vi "MultiChannelfFeedbackCooling (FPGA)_PIDXYZ.vi"() -> ()   [LabVIEW 2016]
doc: "This VI will read single point values from 4 channels of a R Series board at a specified rate."
uses:
  <vilib>/rvi/Emulation/niFpgaGetClockAttributes.vi
  <vilib>/rvi/Emulation/niFpgaSctlEmulationGetInTimedLoop.vi
  <vilib>/rvi/Emulation/niFpgaEmulationReportErrorSimple.vi
  <vilib>/rvi/eio/common/nirviEmuTemplateMethod_errors.vi
  <vilib>/rvi/Memory/Memory_Emulation/nirvimemoryFastEmulation.vi
  <vilib>/rvi/Memory/Memory_Emulation/nirvimemoryEmulation.vi
  <vilib>/rvi/Emulation/niFpgaEmulationIsFPGAContextNoSignature.vi
  <vilib>/rvi/DataTransferAndStorage/Container/Common/niFpgaContainerGetUniqueNameForEmu.vi
  <vilib>/rvi/Emulation/niFpgaProcessEmulError.vi
  <vilib>/rvi/errors/nirviReportUnexpectedCaseInternalError (U32).vi
  <vilib>/rvi/Memory/Memory_Emulation/niFpgaMemoryEmulationCacheClearOnFirstRun.vi
  <vilib>/rvi/Memory/Memory_Emulation/nirvimemoryEmulationManagerCache_MakeExclusive.vi
  <vilib>/rvi/Memory/Memory_Emulation/niFpgaMemoryEmulationValidateCache.vi
  <vilib>/rvi/Memory/Memory_Emulation/nirvimemoryEmulationManagerCache_InsertValue.vi
  <vilib>/Utility/error.llb/Clear Errors.vi
  <vilib>/rvi/Memory/Memory_Emulation/nirvimemoryEmulationManagerCache_ReleaseExclusive.vi
  <vilib>/rvi/Memory/Memory_Emulation/nirvimemoryEmulationManagerCache_GetValue.vi
  <vilib>/rvi/Memory/Memory_Emulation/nirvimemoryEmulationManagerCache_SetValue.vi
  <vilib>/rvi/Emulation/niFpgaSctlEmulationResourceMgr.vi
  <vilib>/rvi/Emulation/niFpgaCriticalErrorInLSC.vi
  <vilib>/eio/EIONode/EIONode.xnode
  <vilib>/rvi/DataTransferAndStorage/Container/XNode/niFpgaContainer.xnode
  <vilib>/rvi/FXPMathLib/FxpInterpret/XNode/nifxpmath_Interpret.xnode
panel:
  in  "EOM_offset":i16
  in  "EOM_seed":u32=4294967295 caption="seed"
  in  "EOM reset":bool caption="reset"
  in  "EOM_threshold":i16
  in  "EOM_amplitude":i16
  in  "hp coeff band imgZ":i32[](array[numeric])=[-850883994, 1909449570, 958518847, -975456236, 2033039520, 1020559395]
  in  "lp coeff band imgZ":i32[](array[numeric])=[-955995012, 2025731616, 1001305, -1023351008, 2092954700, 1034533]
  in  "hp coeff band dZ":i32[](array[numeric])=[-850883994, 1909449570, 958518847, -975456236, 2033039520, 1020559395]
  in  "lp coeff band dZ":i32[](array[numeric])=[-955995012, 2025731616, 1001305, -1023351008, 2092954700, 1034533]
  in  "lp coeff band Z":i32[](array[numeric])=[-955995012, 2025731616, 1001305, -1023351008, 2092954700, 1034533]
  in  "hp coeff band Z":i32[](array[numeric])=[-850883994, 1909449570, 958518847, -975456236, 2033039520, 1020559395]
  in  "lp coeff band Y":i32[](array[numeric])=[-955995012, 2025731616, 1001305, -1023351008, 2092954700, 1034533]
  in  "hp coeff band Y":i32[](array[numeric])=[-850883994, 1909449570, 958518847, -975456236, 2033039520, 1020559395]
  in  "lp coeff band X":i32[](array[numeric])=[-955995012, 2025731616, 1001305, -1023351008, 2092954700, 1034533]
  in  "hp coeff band X":i32[](array[numeric])=[-850883994, 1909449570, 958518847, -975456236, 2033039520, 1020559395]
  in  "dg band dZ":fxp<+/-,24,12>
  in  "dg band imgZ":fxp<+/-,24,12>
  in  "dg band Z":fxp<+/-,24,12>
  in  "dg band Y":fxp<+/-,24,12>
  in  "dg band X":fxp<+/-,24,12>
  in  "lp coeff band X":i32[](array[numeric])=[1008310688, 32715568]
  in  "pg 1":fxp<+/-,24,12>
  in  "ig 1":fxp<+/-,24,6>
  in  "pg 0":fxp<+/-,24,12>
  in  "ig 0":fxp<+/-,24,6>
  in  "pg_img":fxp<+/-,24,12>
  in  "dg_img":fxp<+/-,24,12>
  in  "ig_img":fxp<+/-,24,6>
  in  "setpt_img":i16
  out "AI_img":i16
  in  "lp coeff_img":i32[](array[numeric])=[1008310688, 32715568]
  in  "Upper lim_img":fxp<+/-,16,16>
  in  "Lower lim_img":fxp<+/-,16,16>
  in  "lp coeff d2":i32[](array[numeric])=[1008310688, 32715568]
  in  "hp coeff_img":i32[](array[numeric])=[946630756, 1010186290]
  out "tot_fb_img":i16
  out "fb_img":i16
  in  "output offset_img":i16
  in  "lp coeff 2":i32[](array[numeric])=[1008310688, 32715568]
  in  "data_buffer3":i16
  in  "Arb gain (ch2)":fxp<+/-,24,12>=0.5 caption="RMS"
  in  "lp coeff 0":i32[](array[numeric])=[1008310688, 32715568]
  in  "lp coeff 1":i32[](array[numeric])=[1008310688, 32715568]
  in  "hp coeff d2":i32[](array[numeric])=[946630756, 1010186290]
  in  "hp coeff 2":i32[](array[numeric])=[946630756, 1010186290]
  in  "hp coeff 1":i32[](array[numeric])=[946630756, 1010186290]
  in  "hp coeff 0":i32[](array[numeric])=[946630756, 1010186290]
  in  "Use_PID2_X 2":bool
  out "AI5":i16
  in  "Dc Pos d2":i16
  out "tot_fb_2":i16
  out "tot_fb_1":i16
  out "tot_fb_0":i16
  out "fb_d2":i16
  in  "output offset 2":i16
  in  "output offset 1":i16
  in  "output offset 0":i16
  in  "Lower lim 4":fxp<+/-,16,16>
  in  "Upper lim d0 3":fxp<+/-,16,16>
  in  "pg d0 3":fxp<+/-,24,12>
  in  "ig d03":fxp<+/-,24,6>
  in  "dg d0 3":fxp<+/-,24,12>
  out "fb_2":i16
  in  "ig 3":fxp<+/-,24,6>
  out "written_address":u32
  in  "ready_to_write":bool
  in  "Arb steps per cycle":u16
  in  "data_buffer2":i16
  in  "data_buffer_1":i16
  in  "write_address":u16
  in  "Arb gain (ch1)":fxp<+/-,24,12>=0.5 caption="RMS"
  in  "Arb gain (ch0)":fxp<+/-,24,12>=0.5 caption="RMS"
  out "fb_1":i16
  out "fb_0":i16
  in  "Dc Pos 1":i16
  in  "Dc Pos 0":i16
  in  "Lower lim 2":fxp<+/-,16,16>
  in  "Upper lim 2":fxp<+/-,16,16>
  in  "dg 2":fxp<+/-,24,12>
  in  "pg 2":fxp<+/-,24,12>
  out "AI2":i16
  in  "Dc Pos 2":i16
  out "AI1":i16
  in  "dg 1":fxp<+/-,24,12>
  in  "Upper lim 1":fxp<+/-,16,16>
  in  "Lower lim 1":fxp<+/-,16,16>
  out "AI0":i16
  in  "dg 0":fxp<+/-,24,12>
  in  "Upper lim 0":fxp<+/-,16,16>
  in  "Lower lim 0":fxp<+/-,16,16>
  in  "Count(uSec)":u32
  out "FPGA Error Out":errorcluster
  in  "Stop":bool
  # "test"
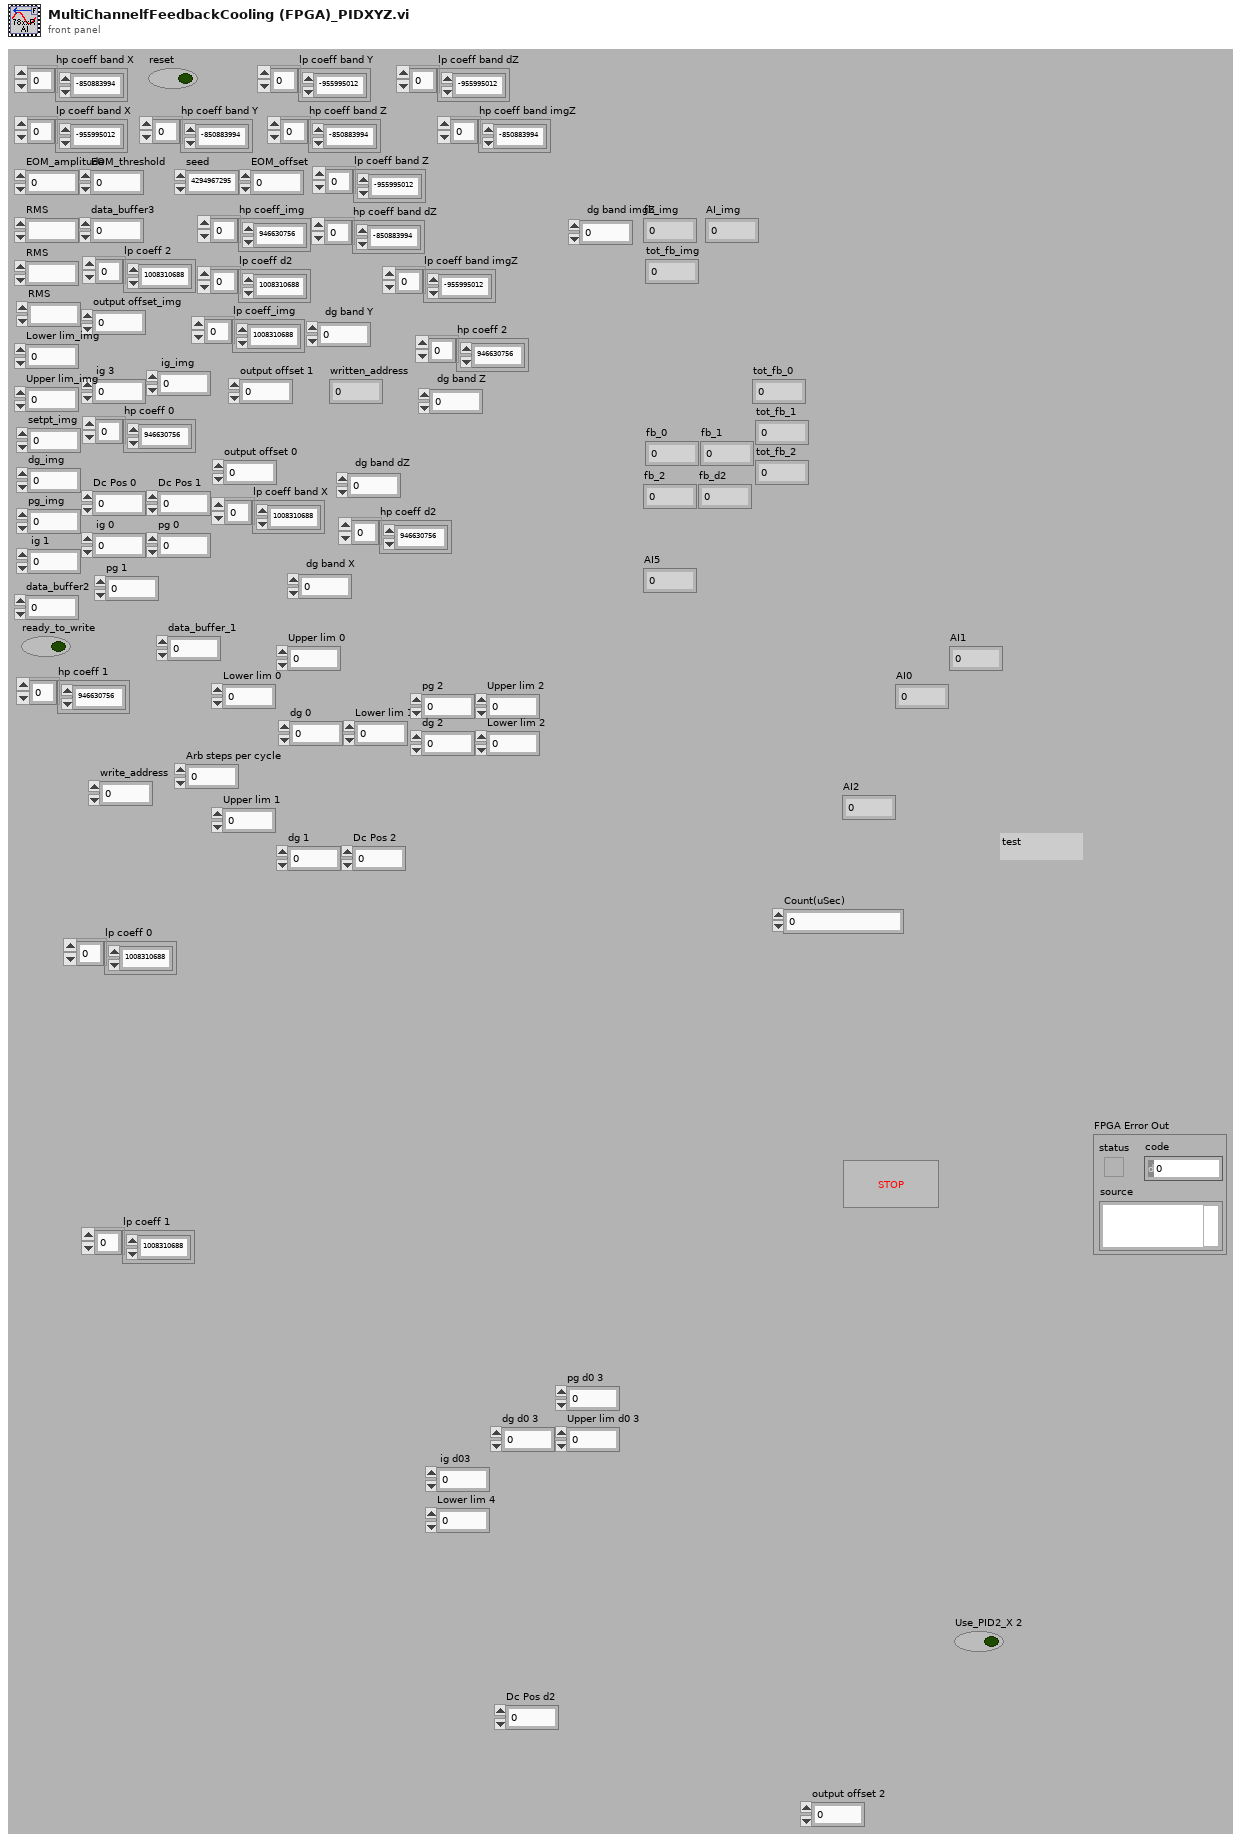
[diagram p1: front panel]
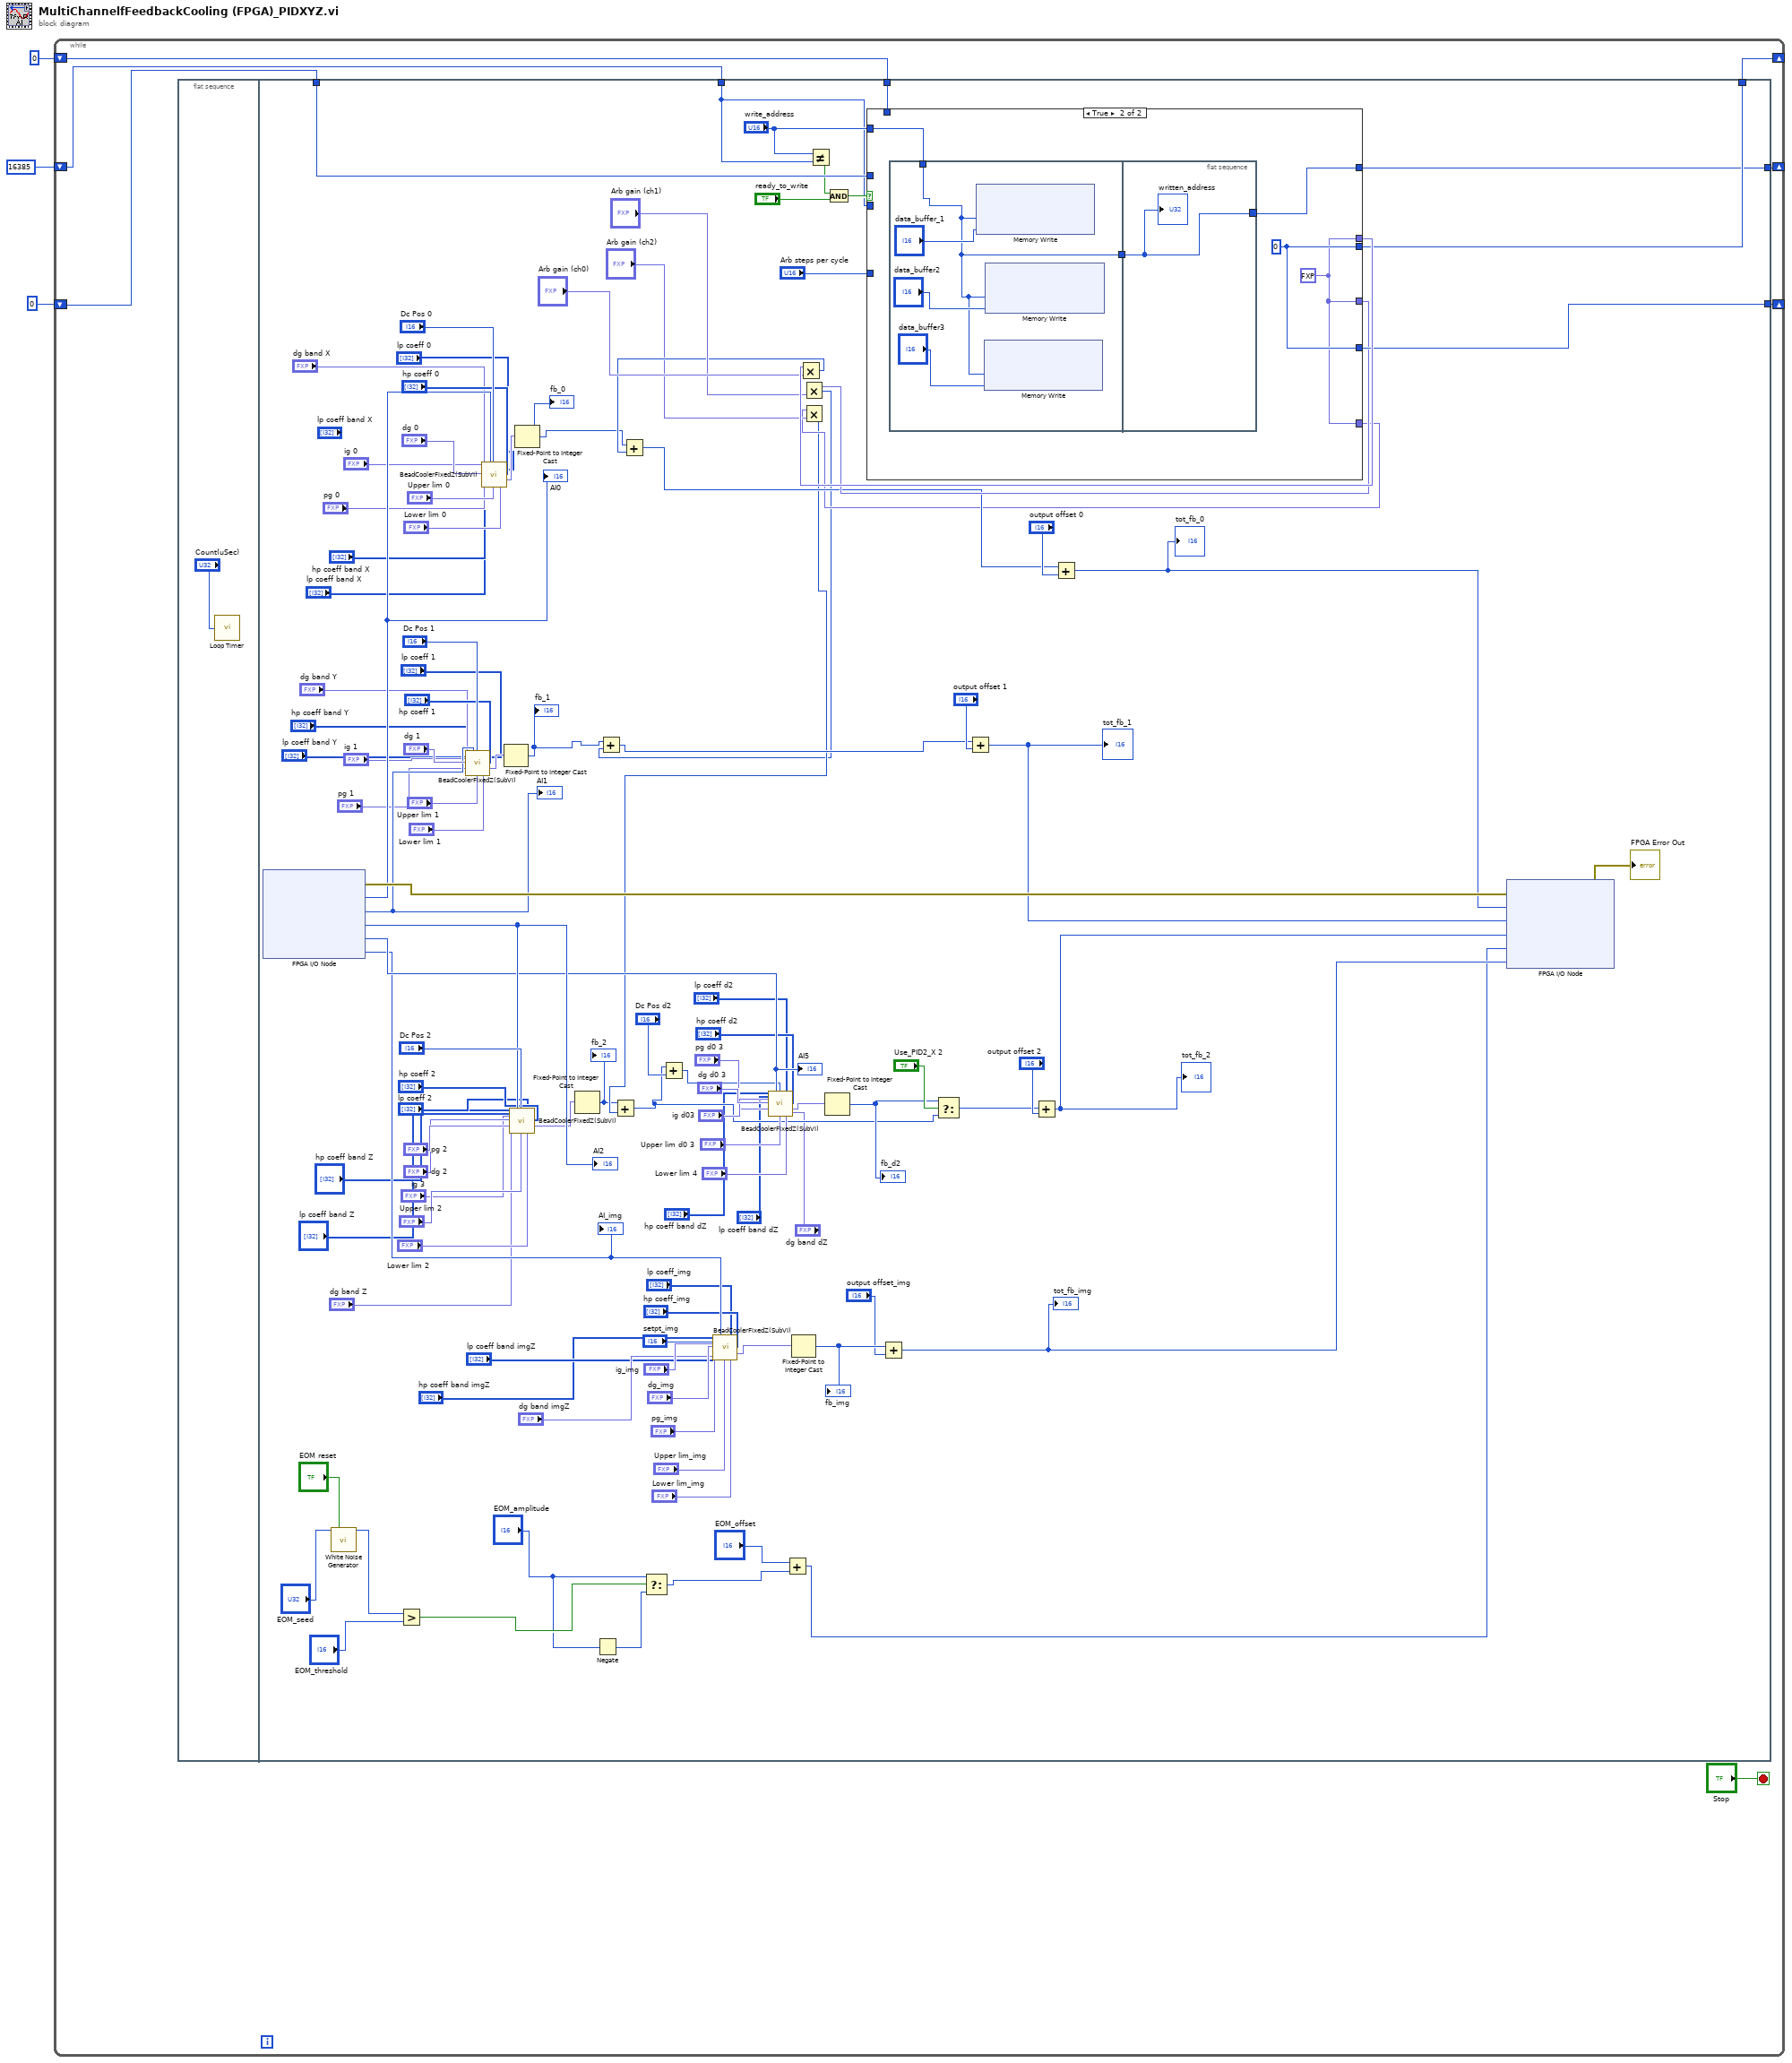
[diagram p0: block diagram]
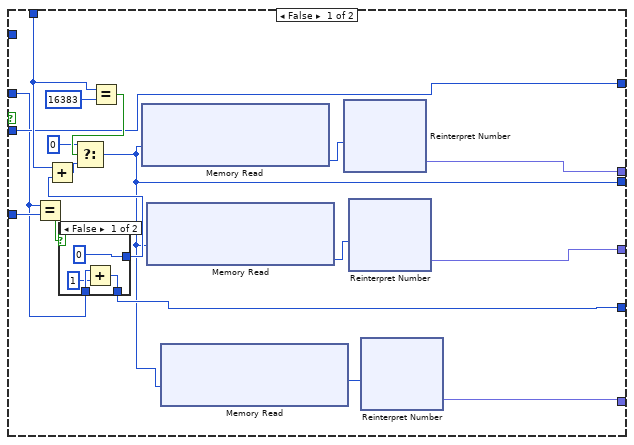
[diagram p2: hidden frame]
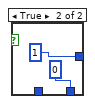
[diagram p3: hidden frame]
diagram:
  n1 = while {
    shift-right: [w9] -> _
    shift-left: u16 0 ("t") -> [w8]
    shift-right: [w7] -> _
    shift-left: u16 0 ("t") -> [w4]
    shift-right: [w6] -> _
    shift-left: u32 16385 ("write_address") -> [w5]
    stop <- "Stop" stop-if-true
    n2 = flat-sequence {
      tunnel: [w110] -> w9
      tunnel: w8 -> [w109]
      tunnel: [w107] -> w7
      tunnel: w4 -> [w106]
      tunnel: [w105] -> w6
      tunnel: w5 -> [w97]
      frame #0 {
        n3 = call "Loop Timer"("Count(uSec)"="Count(uSec)") -> ()  [unwired: 1 out]
      }
      frame #1 {
        n4 = xnode "FPGA I/O Node"() -> ("error out"=w127:errorcluster, "Connector0/AI0"=w96:i16, "Connector0/AI1"=w95:i16, "Connector0/AI2"=w92:i16, "Connector0/AI5"=w80:i16, "Connector0/AI4"=w55:i16)  [unwired: 6 in, 5 out]
        "AI0" <- w96
        "AI1" <- w95
        "AI2" <- w92
        "AI5" <- w80
        "AI_img" <- w55
        n5 = call "White Noise Generator"("seed"="EOM_seed", "reset"="EOM reset") -> ("white noise out"=w21:i16)  [unwired: 13 in]
        n6 = Greater?(x=w21, y="EOM_threshold") -> (0:w19:bool)
        n7 = call "BeadCoolerFixedZ(SubVI).vi"("hp coeff band"="hp coeff band Y", "lp coeff band"="lp coeff band Y", "ig"="ig 1", "dg"="dg 1", "pg"="pg 1", "dg band"="dg band Y", "AI0"=w95, "Dc Pos"="Dc Pos 1", "Upper lim"="Upper lim 1", "lp coeff"="lp coeff 1", "Lower lim"="Lower lim 1", "hp coeff"="hp coeff 1") -> ("Output"=w94:fxp<+/-,16,16>)  [unwired: 15 in]
        n8 = call "BeadCoolerFixedZ(SubVI).vi"("hp coeff band"="hp coeff band X", "lp coeff band"="lp coeff band X", "ig"="ig 0", "dg"="dg 0", "pg"="pg 0", "dg band"="dg band X", "AI0"=w96, "Dc Pos"="Dc Pos 0", "Upper lim"="Upper lim 0", "lp coeff"="lp coeff 0", "Lower lim"="Lower lim 0", "hp coeff"="hp coeff 0") -> ("Output"=w98:fxp<+/-,16,16>)  [unwired: 15 in]
        n9 = Fixed-Point to Integer Cast(1:w94) -> (0:w60:i16)
        "fb_1" <- w60
        n10 = call "BeadCoolerFixedZ(SubVI).vi"("hp coeff band"="hp coeff band Z", "lp coeff band"="lp coeff band Z", "ig"="ig 3", "dg"="dg 2", "pg"="pg 2", "dg band"="dg band Z", "AI0"=w92, "Dc Pos"="Dc Pos 2", "Upper lim"="Upper lim 2", "lp coeff"="lp coeff 2", "Lower lim"="Lower lim 2", "hp coeff"="hp coeff 2") -> ("Output"=w68:fxp<+/-,16,16>)  [unwired: 15 in]
        n11 = Fixed-Point to Integer Cast(1:w98) -> (0:w63:i16)
        "fb_0" <- w63
        n12 = Fixed-Point to Integer Cast(1:w68) -> (0:w22:i16)
        "fb_2" <- w22
        n13 = Negate(x="EOM_amplitude") -> (-x=w17:i16)
        n14 = Select(t="EOM_amplitude", s=w19, f=w17) -> (s? t:f=w13:i16)
        n15 = call "BeadCoolerFixedZ(SubVI).vi"("hp coeff band"="hp coeff band imgZ", "lp coeff band"="lp coeff band imgZ", "ig"="ig_img", "dg"="dg_img", "pg"="pg_img", "dg band"="dg band imgZ", "AI0"=w55, "Dc Pos"="setpt_img", "Upper lim"="Upper lim_img", "lp coeff"="lp coeff_img", "Lower lim"="Lower lim_img", "hp coeff"="hp coeff_img") -> ("Output"=w54:fxp<+/-,16,16>)  [unwired: 15 in]
        n16 = Add(x="EOM_offset", y=w13) -> (x+y=w14:i16)
        n17 = Fixed-Point to Integer Cast(1:w54) -> (0:w53:i16)
        "fb_img" <- w53
        n18 = Not Equal?(x="write_address", y=w97) -> (x != y?=w102:bool)
        n19 = And(x=w102, y="ready_to_write") -> (x .and. y?=w103:bool)
        n20 = case shown="True" w103 {
          tunnel: [w144 w152] -> w112
          tunnel: [w129 w156] -> w110
          tunnel: w109 -> [w137 _]
          tunnel: [w138 w152] -> w100
          tunnel: "Arb steps per cycle" -> [w136 _]
          tunnel: [w131 w156] -> w107
          tunnel: w106 -> [w132 _]
          tunnel: [w135 w154] -> w105
          tunnel: w97 -> [w135 _]
          tunnel: "write_address" -> [_ w153]
          tunnel: [w128 w152] -> w61
          frame False {
            n21 = Equal?(x=w132, y=w136) -> (x = y?=w134:bool)
            n22 = case shown="False" w134 {
              tunnel: [u16 0 ("y") u16 1 ("y")] -> w133
              tunnel: w132 -> [w148 _]
              tunnel: [w146 u16 0] -> w131
              frame False {
                n23 = Add(x=w148, y=u16 1) -> (x+y=w146:u16)
              }
              frame True {
              }
            }
            n24 = Add(x=w137, y=w133) -> (x+y=w140:u16)
            n25 = Equal?(x=w137, y=u16 16383) -> (x = y?=w142:bool)
            n26 = Select(t=u16 0, s=w142, f=w140) -> (s? t:f=w129:u16)
            n27 = xnode ("Memory Read")("Address"=w129) -> ("Data"=w145:i16)  [unwired: 1 in, 1 out]
            n28 = xnode ("Memory Read")("Address"=w129) -> ("Data"=w139:i16)  [unwired: 1 in, 1 out]
            n29 = xnode ("Memory Read")("Address"=w129) -> ("Data"=w130:i16)  [unwired: 1 in, 1 out]
            n30 = xnode "Reinterpret Number"("x"=w145) -> ("y"=w144:fxp<+/-,16,16>)
            n31 = xnode "Reinterpret Number"("x"=w139) -> ("y"=w138:fxp<+/-,16,16>)
            n32 = xnode "Reinterpret Number"("x"=w130) -> ("y"=w128:fxp<+/-,16,16>)
          }
          frame True {
            w156 = u16 0
            w152 = fxp<+/-,16,16> 0.0 ("y")
            n33 = flat-sequence {
              tunnel: [w158] -> w155
              tunnel: w153 -> [w158]
              tunnel: w155 -> [w161]
              tunnel: [w161] -> w154
              frame #0 {
                n34 = xnode ("Memory Write")("Address"=w158, "Data"="data_buffer_1") -> ()  [unwired: 1 in, 1 out]
                n35 = xnode ("Memory Write")("Address"=w158, "Data"="data_buffer3") -> ()  [unwired: 1 in, 1 out]
                n36 = xnode ("Memory Write")("Address"=w158, "Data"="data_buffer2") -> ()  [unwired: 1 in, 1 out]
              }
              frame #1 {
                "written_address" <- w161
              }
            }
          }
        }
        n37 = Multiply(x=w112, y="Arb gain (ch0)") -> (x*y=w84:i16)
        n38 = Add(x=w63, y=w84) -> (x+y=w73:i16)
        n39 = Multiply(x=w100, y="Arb gain (ch1)") -> (x*y=w57:i16)
        n40 = Add(x=w60, y=w57) -> (x+y=w59:i16)
        n41 = Multiply(x=w61, y="Arb gain (ch2)") -> (x*y=w58:i16)
        n42 = Add(x=w22, y=w58) -> (x+y=w67:i16)
        n43 = Add(x=w67, y="Dc Pos d2") -> (x+y=w64:i16)
        n44 = call "BeadCoolerFixedZ(SubVI).vi"("hp coeff band"="hp coeff band dZ", "lp coeff band"="lp coeff band dZ", "ig"="ig d03", "dg"="dg d0 3", "pg"="pg d0 3", "dg band"="dg band dZ", "AI0"=w80, "Dc Pos"=w64, "Upper lim"="Upper lim d0 3", "lp coeff"="lp coeff d2", "Lower lim"="Lower lim 4", "hp coeff"="hp coeff d2") -> ("Output"=w86:fxp<+/-,16,16>)  [unwired: 15 in]
        n45 = Fixed-Point to Integer Cast(1:w86) -> (0:w76:i16)
        "fb_d2" <- w76
        n46 = Add(x=w53, y="output offset_img") -> (x+y=w52:i16)
        "tot_fb_img" <- w52
        n47 = Select(t=w76, s="Use_PID2_X 2", f=w67) -> (s? t:f=w75:i16)
        n48 = Add(x=w59, y="output offset 1") -> (x+y=w77:i16)
        "tot_fb_1" <- w77
        n49 = Add(x=w75, y="output offset 2") -> (x+y=w74:i16)
        "tot_fb_2" <- w74
        n50 = Add(x=w73, y="output offset 0") -> (x+y=w78:i16)
        "tot_fb_0" <- w78
        n51 = xnode "FPGA I/O Node"("error in"=w127, "Connector0/AO0"=w78, "Connector0/AO1"=w77, "Connector0/AO2"=w74, "Connector0/AO3"=w14, "Connector0/AO4"=w52) -> ("error out"=→"FPGA Error Out":errorcluster)  [unwired: 5 in, 5 out]
      }
    }
  }
